vi "swerve_begin.vi"(9 "D":dbl, 10 "I":dbl, 11 "P":dbl) -> (3 "error out":errorcluster)   [LabVIEW 2012]
uses:
  <vilib>/Rock Robotics/WPI/CAN/Jaguar/SubVIs/WPI_CANJaguar_ControlMode.ctl
  <vilib>/Rock Robotics/WPI/CAN/Jaguar/SubVIs/WPI_CANJaguar_BrakeCoastMode.ctl
  <vilib>/Rock Robotics/WPI/CAN/Jaguar/SubVIs/WPI_CANJaguar_SpeedReference.ctl
  <vilib>/Rock Robotics/WPI/MotorControl/WPI_MotorControlOpenCANJaguar.vi
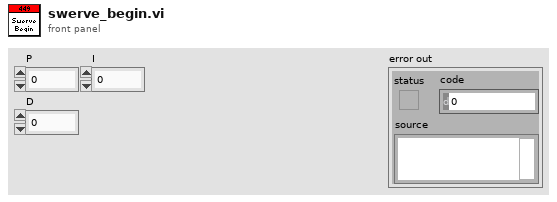
[diagram p1: front panel]
types:
  T1 = typedef "WPI_CANJaguar_SpeedReference.ctl" = u8
  T2 = typedef "WPI_CANJaguar_BrakeCoastMode.ctl" = enum8{"Jumper", "Brake", "Coast"}
  T3 = typedef "WPI_CANJaguar_ControlMode.ctl" = enum8{"Percent VBus", "Current", "Speed", "Position", "Voltage"}
  T4 = typedef "WPI_MotorControlDeviceRef.ctl" = cluster{"DeviceStatus":errorcluster, "Type":enum16{"PWM", "CAN"}, "PWM":cluster{"Digital Module":T5, "PWM Channel":T6, "DeadBand":T7}, "CAN":cluster{"Device Number":u8, "Control Mode":T3, "Semaphore":T8, "Max Vout":dbl}, "Invert":bool, "TransformRef":T9, "InvTransformRef":T9}
  T5 = typedef "FPGA_TypedefDigitalModule.ctl" = enum16{"Digital Module 1", "Digital Module 2"}
  T6 = typedef "FPGA_DIOPWMChannel.ctl" = enum8{"PWM 1", "PWM 2", "PWM 3", "PWM 4", "PWM 5", "PWM 6", "PWM 7", "PWM 8", "PWM 9", "PWM 10", "Invalid"}
  T7 = typedef "WPI_PWMDeadband.ctl" = cluster{"Name":string, "maxPositivePwm":i32, "minPositivePwm":i32, "centerPwm":i32, "maxNegativePwm":i32, "minNegativePwm":i32, "angularRange":u16}
  T8 = typedef "Semaphore RefNum" = refnum<k1>
  T9 = typedef "WPI_PWMTransform_ConPane.ctl" = refnum<vi>
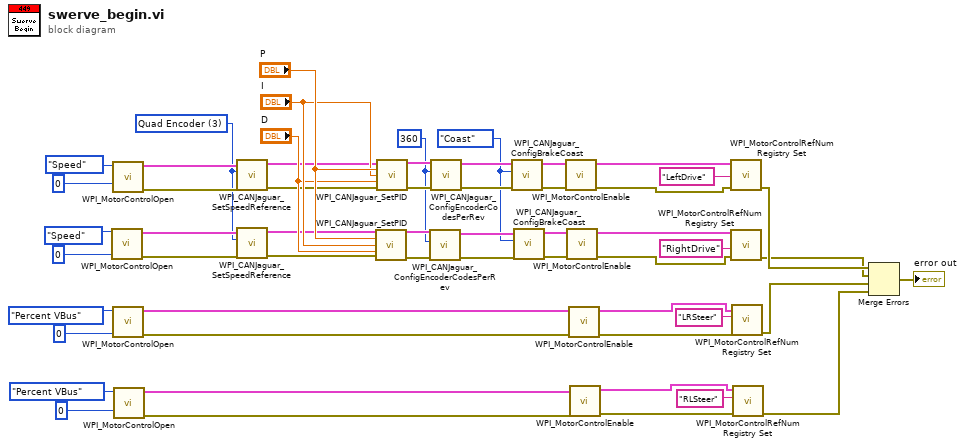
[diagram p0: block diagram]
diagram:
  w10 = T1 3 items=["Encoder"=0, "Inv Encoder"=2, "Quad Encoder"=3, "None"=255] ("Speed Reference")
  w31 = WPI_CANJaguar_BrakeCoastMode."Coast" ("Brake / Coast Mode")
  w36 = u16 360 ("Encoder Codes Per Rev")
  n1 = call-poly <vilib>:"WPI_MotorControlOpen.vi"("Device Number"=u8 0, "Control Mode"=WPI_CANJaguar_ControlMode."Speed") -> ("error out"=w11:errorcluster, "MotorControlDeviceRef"=w14:T4)  [unwired: 8 in]
  n2 = call-poly <vilib>:"WPI_MotorControlOpen.vi"("Device Number"=u8 0, "Control Mode"=WPI_CANJaguar_ControlMode."Speed") -> ("error out"=w16:errorcluster, "MotorControlDeviceRef"=w18:T4)  [unwired: 8 in]
  n3 = call-poly <vilib>:"WPI_MotorControlOpen.vi"("Device Number"=u8 0, "Control Mode"=WPI_CANJaguar_ControlMode."Percent VBus") -> ("error out"=w20:errorcluster, "MotorControlDeviceRef"=w22:T4)  [unwired: 8 in]
  n4 = call-poly <vilib>:"WPI_MotorControlOpen.vi"("Device Number"=u8 0, "Control Mode"=WPI_CANJaguar_ControlMode."Percent VBus") -> ("error out"=w19:errorcluster, "MotorControlDeviceRef"=w21:T4)  [unwired: 8 in]
  n5 = call <vilib>:"WPI_CANJaguar_SetSpeedReference.vi"("error in (no error)"=w16, "Speed Reference"=w10, "CAN Jaguar Ref"=w18) -> ("error out"=w15:errorcluster, "CAN Jaguar Ref Out"=w17:T4)  [unwired: 7 in]
  n6 = call <vilib>:"WPI_CANJaguar_SetSpeedReference.vi"("error in (no error)"=w11, "Speed Reference"=w10, "CAN Jaguar Ref"=w14) -> ("error out"=w12:errorcluster, "CAN Jaguar Ref Out"=w13:T4)  [unwired: 7 in]
  n7 = call <vilib>:"WPI_CANJaguar_SetPID.vi"("CAN Jaguar Ref"=w13, "P"="P", "I"="I", "D"="D", "error in (no error)"=w12) -> ("CAN Jaguar Ref Out"=w42:T4, "error out"=w41:errorcluster)  [unwired: 9 in]
  n8 = call <vilib>:"WPI_CANJaguar_SetPID.vi"("CAN Jaguar Ref"=w17, "P"="P", "I"="I", "D"="D", "error in (no error)"=w15) -> ("CAN Jaguar Ref Out"=w43:T4, "error out"=w44:errorcluster)  [unwired: 9 in]
  n9 = call <vilib>:"WPI_CANJaguar_ConfigEncoderCodesPerRev.vi"("error in (no error)"=w41, "Encoder Codes Per Rev"=w36, "CAN Jaguar Ref"=w42) -> ("error out"=w39:errorcluster, "CAN Jaguar Ref Out"=w40:T4)  [unwired: 7 in]
  n10 = call <vilib>:"WPI_CANJaguar_ConfigEncoderCodesPerRev.vi"("error in (no error)"=w44, "Encoder Codes Per Rev"=w36, "CAN Jaguar Ref"=w43) -> ("error out"=w37:errorcluster, "CAN Jaguar Ref Out"=w38:T4)  [unwired: 7 in]
  n11 = call <vilib>:"WPI_CANJaguar_ConfigBrakeCoast.vi"("error in (no error)"=w37, "Brake / Coast Mode"=w31, "CAN Jaguar Ref"=w38) -> ("error out"=w28:errorcluster, "CAN Jaguar Ref Out"=w35:T4)  [unwired: 7 in]
  n12 = call <vilib>:"WPI_CANJaguar_ConfigBrakeCoast.vi"("error in (no error)"=w39, "Brake / Coast Mode"=w31, "CAN Jaguar Ref"=w40) -> ("error out"=w30:errorcluster, "CAN Jaguar Ref Out"=w33:T4)  [unwired: 7 in]
  n13 = call <vilib>:"WPI_MotorControlEnable.vi"("error in (no error)"=w28, "CAN Jaguar Ref"=w35) -> ("error out"=w27:errorcluster, "CAN Jaguar Ref Out"=w34:T4)  [unwired: 8 in]
  n14 = call <vilib>:"WPI_MotorControlEnable.vi"("error in (no error)"=w30, "CAN Jaguar Ref"=w33) -> ("error out"=w29:errorcluster, "CAN Jaguar Ref Out"=w32:T4)  [unwired: 8 in]
  n15 = call <vilib>:"WPI_MotorControlEnable.vi"("error in (no error)"=w20, "CAN Jaguar Ref"=w22) -> ("error out"=w26:errorcluster, "CAN Jaguar Ref Out"=w25:T4)  [unwired: 8 in]
  n16 = call <vilib>:"WPI_MotorControlEnable.vi"("error in (no error)"=w19, "CAN Jaguar Ref"=w21) -> ("error out"=w24:errorcluster, "CAN Jaguar Ref Out"=w23:T4)  [unwired: 8 in]
  n17 = call <vilib>:"WPI_MotorControlRefNum Registry Set.vi"("error in (no error)"=w27, "refnum name"="LeftDrive", "MotorControlDevRef"=w34) -> ("error out"=w9:errorcluster)  [unwired: 7 in, 1 out]
  n18 = call <vilib>:"WPI_MotorControlRefNum Registry Set.vi"("error in (no error)"=w29, "refnum name"="RightDrive", "MotorControlDevRef"=w32) -> ("error out"=w8:errorcluster)  [unwired: 7 in, 1 out]
  n19 = call <vilib>:"WPI_MotorControlRefNum Registry Set.vi"("error in (no error)"=w26, "refnum name"="LRSteer", "MotorControlDevRef"=w25) -> ("error out"=w7:errorcluster)  [unwired: 7 in, 1 out]
  n20 = call <vilib>:"WPI_MotorControlRefNum Registry Set.vi"("error in (no error)"=w24, "refnum name"="RLSteer", "MotorControlDevRef"=w23) -> ("error out"=w6:errorcluster)  [unwired: 7 in, 1 out]
  n21 = Merge Errors(w9, w8, w7, w6) -> (→"error out":errorcluster)
